vi "throw configuration load error.vi"(7 "source":string="throw configuration load error.vi", 8 "error in":errorcluster) -> (0 "error out":errorcluster)   [LabVIEW 2013, in "TBM module configuration.lvclass"]
doc: "Converts a specific error into a generic configuration error. This error makes it so people can expect a specific code when a module fails to load, but then the actual issue can be recovered later."
uses:
  TBM module configuration.lvclass
  <vilib>/NI/Configuration Framework/NISE_CEF_TreeControl.lvlib
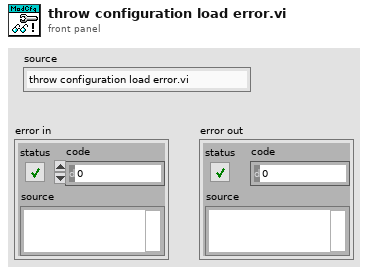
[diagram p1: front panel]
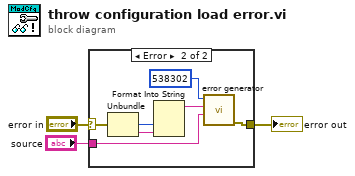
[diagram p0: block diagram]
diagram:
  n1 = case shown="Error" "error in" {
    selector: "error in" -> [w4 w9]
    tunnel: [w4 w10] -> w3
    tunnel: "source" -> [_ w5]
    frame No Error {
    }
    frame Error {
      n2 = Unbundle(w9) -> ("code"=w8:i32, "source"=w7:string)  [unwired: 1 out]
      n3 = Format Into String(w8, w7) -> (resulting string=w6:string)  [unwired: 3 in, 1 out]
      n4 = call <vilib>:"error generator.vi"("source"=w5, "append error message"=w6, "error code (0)"=538302) -> ("error out"=w10:errorcluster)  [unwired: 6 in]
    }
  }
  "error out" <- w3
